vi "Weather Station UI_EX.vi"() -> ()   [LabVIEW 2021]
doc: "This is the main VI in the Weather Station project. It contains the user interface for a temperature warning system. Temperature is retrieved every half second; data is logged when a warning has occurred."
uses:
  WeatherData.ctl
  WeatherStationState.ctl
  Instance           2 26Saved   Weather Station UI .vi
panel:
  out "Warning":string
  in  "Lower Limit":dbl=20.0
  in  "Upper Limit":dbl=30.0
  in  "Stop Button":bool
  out "Temperature History":dbl(graph)
  # "Temperature Ranges (C)"
  # "Freeze"
  # "Heat \nStroke"
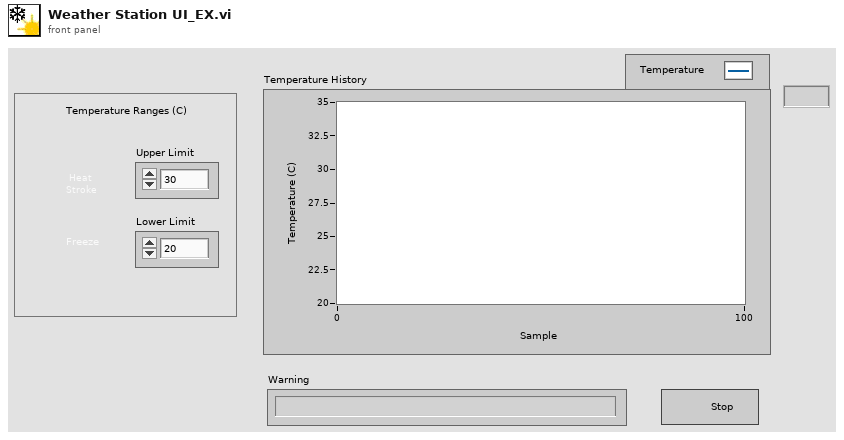
[diagram p1: front panel]
types:
  T1 = typedef "WeatherStationState.ctl" = enum16{"Acquisition", "Analysis", "Data Log", "Time Check"}
  T2 = typedef "WeatherData.ctl" = cluster{"Current Temperature":dbl, "Max Temperature":dbl, "Min Temperature":dbl, "Warning?":bool, "Warning Text":string}
  T3 = enum16{"open", "replace", "create", "open or create", "replace or create", "replace or create with confirmation"}
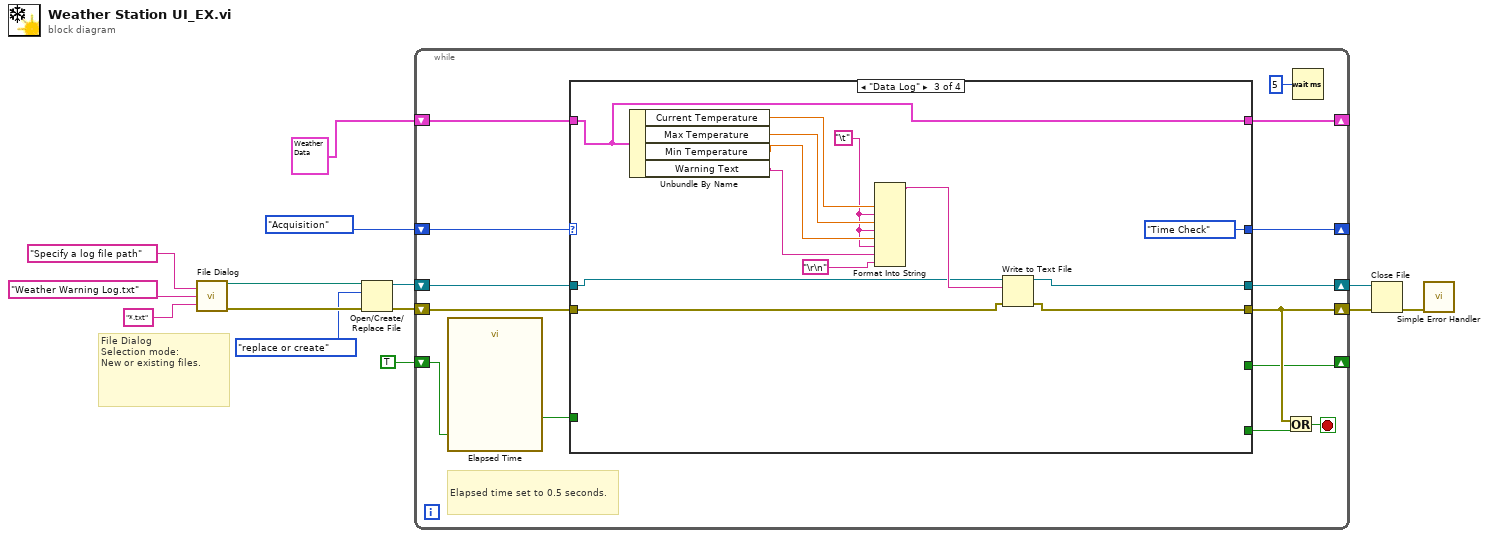
[diagram p0: block diagram]
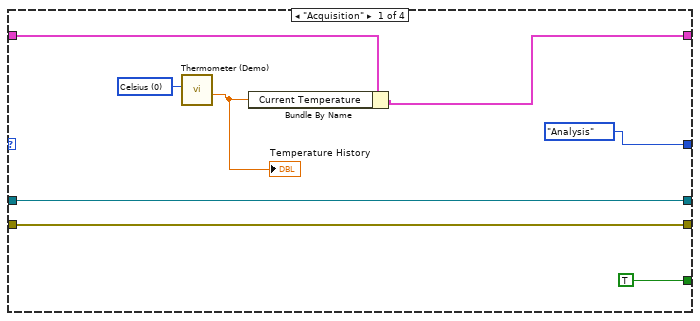
[diagram p2: hidden frame]
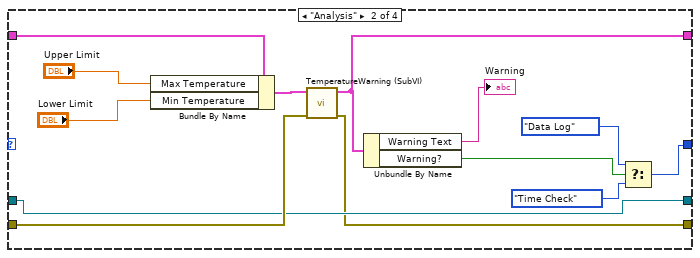
[diagram p3: hidden frame]
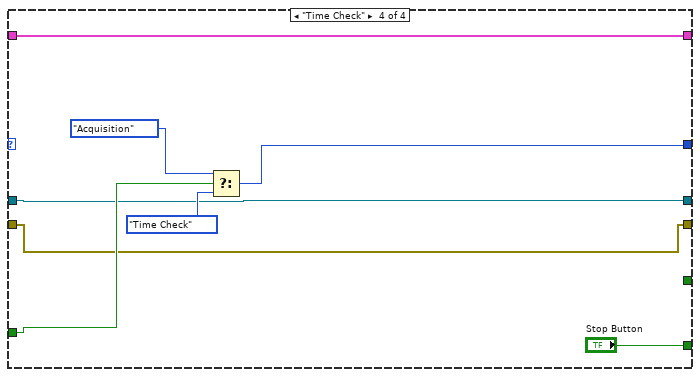
[diagram p4: hidden frame]
diagram:
  # "File Dialog\nSelection mode:\nNew or existing files."
  n1 = call "File Dialog"("prompt"="Specify a log file path", "default name"="Weather Warning Log.txt", "pattern (all files)"="*.txt" ("pattern label")) -> ("selected path"=w8:path, "error out"=w5:errorcluster)  [unwired: 9 in, 2 out]
  n2 = Open/Create/Replace File(file path (use dialog)=w8, error in=w5, operation (0:open)=T3."replace or create") -> (refnum out=w10:refnum<file>, error out=w9:errorcluster)  [unwired: 3 in, 1 out]
  n3 = while {
    shift-right: [w21] -> w14
    shift-left: w9 -> [w28]
    shift-right: [w26] -> w13
    shift-left: w10 -> [w25]
    shift-right: [w16] -> _
    shift-left: TRUE ("stop") -> [w23]
    shift-right: [w18] -> _
    shift-left: T2 {"Current Temperature"=0.0, "Max Temperature"=0.0, "Min Temperature"=0.0, "Warning?"=FALSE, "Warning Text"="No Warning"} ("Cluster") -> [w19]
    shift-right: [w17] -> _
    shift-left: WeatherStationState."Acquisition" ("Enum") -> [w20]
    stop <- w27 stop-if-true
    # "Elapsed time set to 0.5 seconds."
    n4 = call "Elapsed Time"("Reset"=w23) -> ("Time has Elapsed"=w22:bool)  [unwired: 11 in, 7 out]
    n5 = case shown="\"Data Log\"" w20 {
      tunnel: [w35 w38 w55 w64] -> w21
      tunnel: w28 -> [w35 w45 w56 w64]
      tunnel: [w36 w39 w57 w65] -> w26
      tunnel: w25 -> [w36 w39 w58 w65]
      tunnel: w22 -> [_ _ _ w70]
      tunnel: w19 -> [w32 w49 w53 w66]
      tunnel: [w29 w37 w53 w66] -> w18
      tunnel: [WeatherStationState."Analysis" ("Enum") w40 WeatherStationState."Time Check" ("Enum") w67] -> w17
      tunnel: [TRUE _ _ _] -> w16
      tunnel: [_ _ _ "Stop Button"] -> w15
      frame "Acquisition" {
        w34 = u16 0 items=["Celsius", "Fahrenheit"] ("Units (0: Celsius)")
        n6 = call "Thermometer (Demo).vi"("Units (0: Celsius)"=w34) -> ("Temperature Value"=w33:dbl)  [unwired: 10 in]
        "Temperature History" <- w33
        n7 = Bundle By Name(cluster=w32, "Current Temperature"=w33) -> (w29:T2)
      }
      frame "Analysis" {
        n8 = Bundle By Name(cluster=w49, "Max Temperature"="Upper Limit", "Min Temperature"="Lower Limit") -> (w46:T2)
        n9 = call "TemperatureWarning (SubVI).vi"("error in (no error)"=w45, "Weather In"=w46) -> ("error out"=w38:errorcluster, "Weather Out"=w37:T2)  [unwired: 8 in]
        n10 = Unbundle By Name(w37) -> ("Warning Text"=→"Warning":string, "Warning?"=w43:bool)
        n11 = Select(t=WeatherStationState."Data Log" ("Enum"), s=w43, f=WeatherStationState."Time Check" ("Enum")) -> (s? t:f=w40:T1)
      }
      frame "Data Log" {
        w50 = "\t"
        n12 = Unbundle By Name(w53) -> ("Current Temperature"=w62:dbl, "Max Temperature"=w61:dbl, "Min Temperature"=w60:dbl, "Warning Text"=w52:string)
        n13 = Format Into String(w62, w50, w61, w50, w60, w50, w52, "\r\n") -> (resulting string=w59:string)  [unwired: 3 in, 1 out]
        n14 = Write to Text File(file (use dialog)=w58, text=w59, error in=w56) -> (refnum out=w57:refnum<file>, error out=w55:errorcluster)  [unwired: 1 in, 1 out]
      }
      frame "Time Check" {
        n15 = Select(t=WeatherStationState."Acquisition" ("Enum"), s=w70, f=WeatherStationState."Time Check") -> (s? t:f=w67:T1)
      }
    }
    n16 = Or(x=w21, y=w15) -> (x .or. y?=w27:bool)
    n17 = Wait (ms)(milliseconds to wait=u32 5 ("y")) -> ()  [unwired: 1 out]
  }
  n18 = Close File(refnum=w13, error in=w14) -> (error out=w12:errorcluster)  [unwired: 1 out]
  n19 = call <vilib>:"Simple Error Handler.vi"("error in (no error)"=w12) -> ()  [unwired: 4 in, 5 out]
